vi "数组的最大值与最小值.vi"() -> ()   [LabVIEW 2018]
panel:
  in  "停止":bool
  out "最小值":dbl
  out "最小索引":i32[](array[numeric])
  out "最大索引":i32[](array[numeric])
  out "最大值":dbl
  in  "数组":dbl[][](array[numeric])
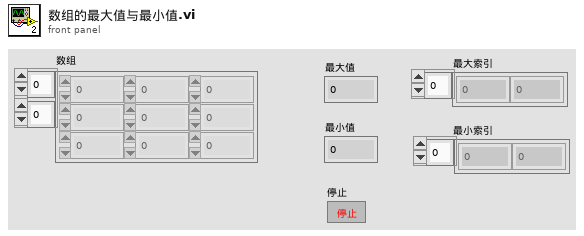
[diagram p1: front panel]
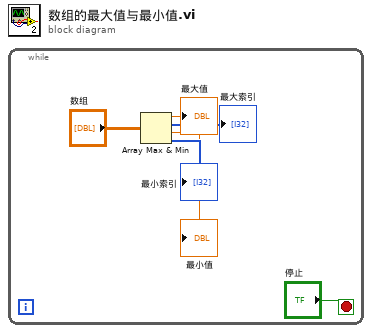
[diagram p0: block diagram]
diagram:
  n1 = while {
    stop <- "停止" stop-if-true
    n2 = Array Max & Min(array="数组") -> (max value=→"最大值":dbl, max index (indices)=→"最大索引":i32[], min value=→"最小值":dbl, min index (indices)=→"最小索引":i32[])
  }
